vi "雷射_FGV.vi"(7 "Enum":T1(ring)=enum."雷射觸發", 8 "error in":errorcluster, 9 "PROGRAM":enum16{"0000", "0002"}(ring), 10 "命令字串":string="RE", 11 "VISA resource name":refnum<visa-resource-name>) -> (0 "error out":errorcluster, 2 "回復訊息":string, 3 "VISA resource name out":refnum<visa-resource-name>)   [LabVIEW 2015]
uses:
  <vilib>/Instr/_visa.llb/VISA Configure Serial Port (Instr).vi
panel:
  in  "Error Table":string[][](table)=[["雷射通訊初始化異常!"], ["雷射未準備就緒!"], ["雷射觸發失敗!"], ["雷射通訊關閉異常!"], ["雷射XY座標值讀"], ["雷射XY座標值寫入異常!"], ["請求雷射程式編號prog#異常!"], ["開起雷射導向光異常!"], ["關閉雷射導向光異常!"]]
  out "substring":string
  out "after substring":string
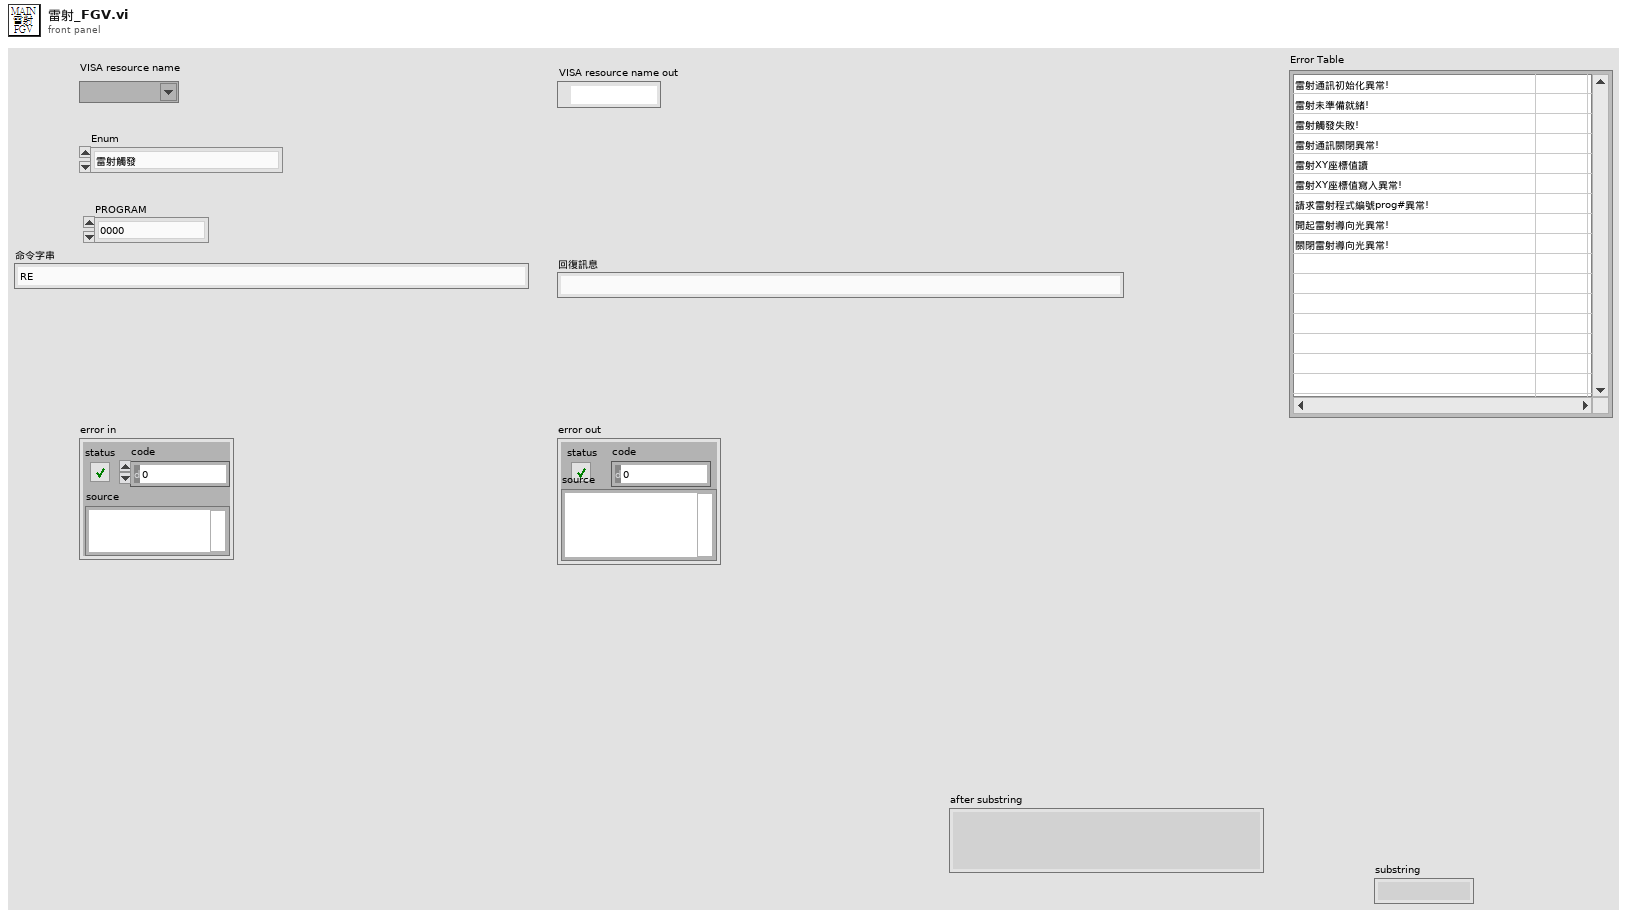
[diagram p1: front panel]
types:
  T1 = enum16{"RS232_Init ", "雷射準備訊號", "雷射觸發", "RS232_Close", "寫入雷射XY座標值與角度", "請求程式編號prog所有資訊", "開起導向光", "關閉導向光", "運行切換"}
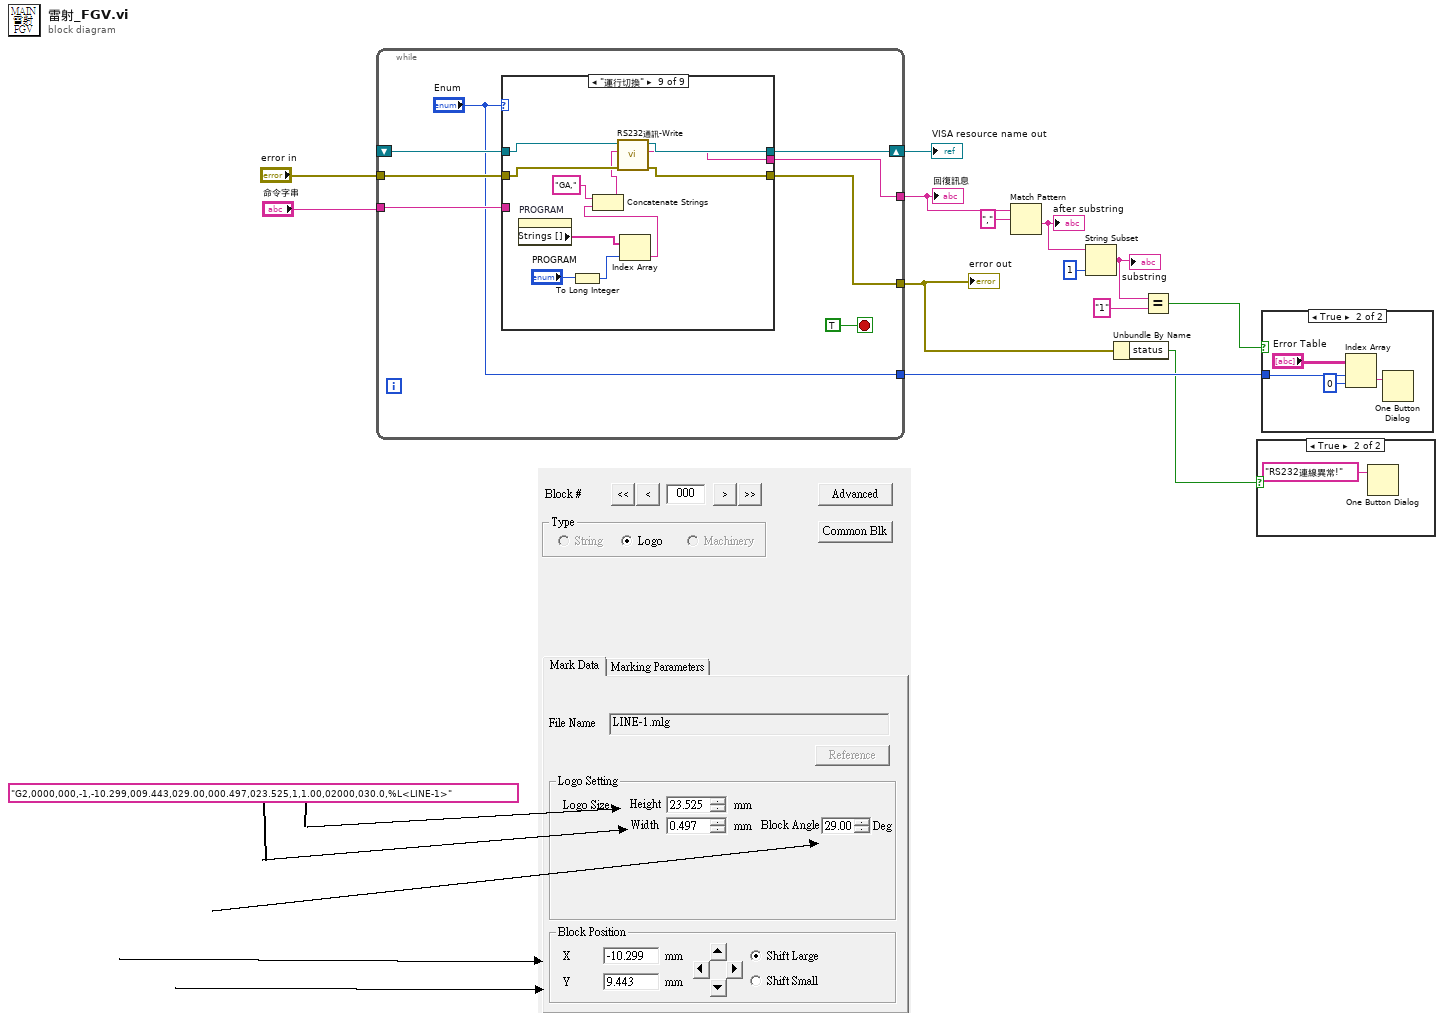
[diagram p0: block diagram]
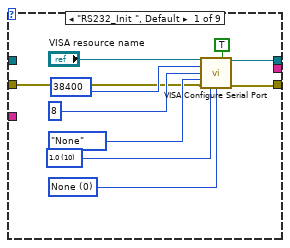
[diagram p4: hidden frame]
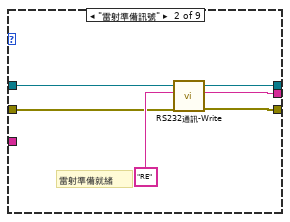
[diagram p5: hidden frame]
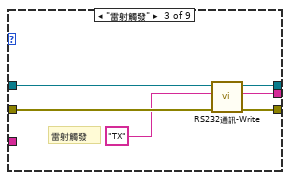
[diagram p6: hidden frame]
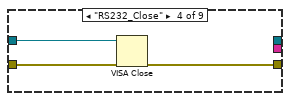
[diagram p7: hidden frame]
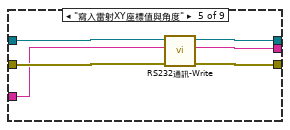
[diagram p8: hidden frame]
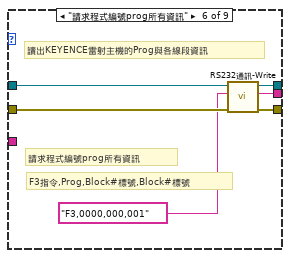
[diagram p9: hidden frame]
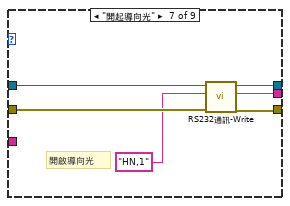
[diagram p10: hidden frame]
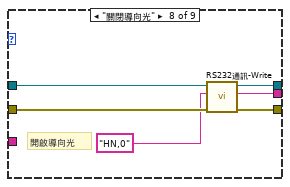
[diagram p11: hidden frame]
diagram:
  (unwired) "G2,0000,000,-1,-10.299,009.443,029.00,000.497,023.525,1,1.00,02000,030.0,%L<LINE-1>"
  n1 = while {
    shift-right: [w17] -> w4
    shift-left: _ -> [w20]
    tunnel: [w16] -> w12
    tunnel: "error in" -> [w19]
    tunnel: [w15] -> w3
    tunnel: "命令字串" -> [w18]
    tunnel: ["Enum"] -> w6
    stop <- TRUE stop-if-true
    n2 = case shown="\"運行切換\"" "Enum" {
      tunnel: [w26 w34 w43 _ w52 w57 w63 w69 w78] -> w17
      tunnel: w20 -> [_ w33 w38 w46 w51 w58 w64 w70 w79]
      tunnel: w19 -> [w24 w32 w40 w44 w50 w54 w60 w66 w81]
      tunnel: [w23 w35 w41 w45 w49 w55 w61 w67 w80] -> w15
      tunnel: w18 -> [_ _ _ _ w47 _ _ _ _]
      tunnel: [_ w37 w42 _ w48 w56 w62 w68 w77] -> w16
      frame "RS232_Init ", Default {
        w31 = u16 0 items=["None", "XON/XOFF", "RTS/CTS", "XON/XOFF & RTS/CTS", "DTR/DSR", "XON/XOFF & DTR/DSR"] ("flow control (0:none)")
        w30 = u16 10 items=["1.0"=10, "1.5"=15, "2.0"=20] ("stop bits (10: 1 bit)")
        n3 = call-poly "VISA Configure Serial Port"("VISA resource name"="VISA resource name", "Enable Termination\nChar (T)"=TRUE ("Enable Termination\nChar (T)"), "baud rate (9600)"=u32 38400, "data bits (8)"=u16 8, "parity (0:none)"=enum16{"None", "Odd", "Even", "Mark", "Space"}."None", "error in (no error)"=w24, "stop bits (10: 1 bit)"=w30, "flow control (0:none)"=w31) -> ("VISA resource name out"=w26:refnum<visa-resource-name>, "error out"=w23:errorcluster)  [unwired: 6 in]
      }
      frame "雷射準備訊號" {
        # "雷射準備就緒"
        n4 = call "RS232通訊-Write.vi"("error in (no error)"=w32, "string"="RE", "VISA Refnum in"=w33) -> ("error out"=w35:errorcluster, "read buffer"=w37:string, "VISA resource name out"=w34:refnum<visa-resource-name>)  [unwired: 6 in]
      }
      frame "雷射觸發" {
        # "雷射觸發"
        n5 = call "RS232通訊-Write.vi"("error in (no error)"=w40, "string"="TX", "VISA Refnum in"=w38) -> ("error out"=w41:errorcluster, "read buffer"=w42:string, "VISA resource name out"=w43:refnum<visa-resource-name>)  [unwired: 6 in]
      }
      frame "RS232_Close" {
        n6 = VISA Close(VISA resource name=w46, error in (no error)=w44) -> (error out=w45:errorcluster)
      }
      frame "寫入雷射XY座標值與角度" {
        n7 = call "RS232通訊-Write.vi"("error in (no error)"=w50, "string"=w47, "VISA Refnum in"=w51) -> ("error out"=w49:errorcluster, "read buffer"=w48:string, "VISA resource name out"=w52:refnum<visa-resource-name>)  [unwired: 6 in]
      }
      frame "請求程式編號prog所有資訊" {
        # "讀出KEYENCE雷射主機的Prog與各線段資訊"
        # "F3指令,Prog,Block#標號,Block#標號"
        # "請求程式編號prog所有資訊"
        n8 = call "RS232通訊-Write.vi"("error in (no error)"=w54, "string"="F3,0000,000,001", "VISA Refnum in"=w58) -> ("error out"=w55:errorcluster, "read buffer"=w56:string, "VISA resource name out"=w57:refnum<visa-resource-name>)  [unwired: 6 in]
      }
      frame "開起導向光" {
        # "開啟導向光"
        n9 = call "RS232通訊-Write.vi"("error in (no error)"=w60, "string"="HN,1", "VISA Refnum in"=w64) -> ("error out"=w61:errorcluster, "read buffer"=w62:string, "VISA resource name out"=w63:refnum<visa-resource-name>)  [unwired: 6 in]
      }
      frame "關閉導向光" {
        # "開啟導向光"
        n10 = call "RS232通訊-Write.vi"("error in (no error)"=w66, "string"="HN,0", "VISA Refnum in"=w70) -> ("error out"=w67:errorcluster, "read buffer"=w68:string, "VISA resource name out"=w69:refnum<visa-resource-name>)  [unwired: 6 in]
      }
      frame "運行切換" {
        n11 = property on="PROGRAM" class="Enum (strict)"() -> ("Strings []"=w76:string[])  [unwired: 2 in, 2 out]
        n12 = To Long Integer(number="PROGRAM") -> (32bit integer=w74:i32)
        n13 = Index Array(array=w76, index=w74) -> (element=w72:string)
        n14 = Concatenate Strings("GA," ("string"), w72) -> (w71:string)
        n15 = call "RS232通訊-Write.vi"("error in (no error)"=w81, "string"=w71, "VISA Refnum in"=w79) -> ("error out"=w80:errorcluster, "read buffer"=w77:string, "VISA resource name out"=w78:refnum<visa-resource-name>)  [unwired: 6 in]
      }
    }
  }
  "回復訊息" <- w12
  "VISA resource name out" <- w4
  "error out" <- w3
  n16 = Match Pattern(string=w12, regular expression=",") -> (after substring=w10:string)  [unwired: 1 in, 3 out]
  "after substring" <- w10
  n17 = String Subset(string=w10, length (rest)=1 ("length (rest)")) -> (substring=w8:string)  [unwired: 1 in]
  "substring" <- w8
  n18 = Unbundle By Name(w3) -> ("status"=w1:bool)
  n19 = Equal?(x=w8, y="1") -> (x = y?=w2:bool)
  n20 = case shown="True" w1 {
    frame False {
    }
    frame True {
      n21 = One Button Dialog(message="RS232連線異常!") -> ()  [unwired: 1 in, 1 out]
    }
  }
  n22 = case shown="True" w2 {
    tunnel: w6 -> [_ w84]
    frame False {
    }
    frame True {
      n23 = Index Array(array="Error Table", index (row)=w84, index (col)=0 ("disabled index (col)")) -> (element=w85:string)
      n24 = One Button Dialog(message=w85) -> ()  [unwired: 1 in, 1 out]
    }
  }
